vi "Send to DAQ - Core.vi"(6 "Timeout (ms)":i32=10000, 8 "error in (no error)":errorcluster, 9 "DAQ Message":T1, 10 "DAQ Address":cluster{"Port":u16, "Path":string}, 11 "DAQ Communication":refnum<class "DAQ Communication.lvclass">) -> (0 "error out":errorcluster)   [LabVIEW 2020, in "DAQ Sender.lvlib" / "DAQ Sender.lvclass"]
doc: "Use this VI to send data to the DAQ. If an entire file is needed to be sent, set File?=True and provide the path of the file to be sent in the Data field. DO NOT USE this VI from inside a uService."
uses:
  DAQ Sender.lvclass
  Interfaces/DAQ Communication/DAQ Communication.lvclass
  Interfaces/DAQ Communication/DAQ Message.ctl
  Ancestor/Ancestor/Ancestor.lvclass/Ancestor.ctl
  Support VIs/Circus Config Param - Core.vi
  Support VIs/Generate Error.vi
  Support VIs/Circus Root Path.vi
  FGV/Error Memory/Get Error Description.vi
  Support VIs/Get PC name.vi
  Ancestor/Ancestor/Read ID.vi
  Support VIs/Get Class Name.vi
  <vilib>/Utility/error.llb/Clear Errors.vi
  FGV/Error Memory/Error Memory Core.vi
  <vilib>/AdvancedString/Delimited String to 1D String Array.vi
  FGV/Error Memory/Error Crt Lvl checker.vi
  FGV/Error Memory/Error Memory Core.vi/40c8088d-b597-4017-91af-faa98e00292e.vi
  FGV/Error Memory/Error Memory Core.vi/d4a3ab98-063c-4e44-b43d-fbdcfe6c2be2.vi
  Support VIs/Global Constants.vi
  Support VIs/Global Memory.vi
  <vilib>/Utility/LVClass/Get LV Class Name.vi
  Support VIs/Is in Packed Library.vi
  Support VIs/TALOS Root path.vi
  Support VIs/Read CSV worksheet.vi
  <vilib>/Utility/error.llb/General Error Handler.vi
  <vilib>/Utility/config.llb/Open Config Data.vi
  <vilib>/Utility/config.llb/Get Section Names.vi
  <vilib>/Utility/config.llb/Get Key Names.vi
  <vilib>/Utility/config.llb/Read Key.vi
  <vilib>/Utility/config.llb/Read Key (String).vi
  <vilib>/Utility/config.llb/Close Config Data.vi
  Support VIs/Error Log.vi
  Ancestor/Ancestor/Ancestor.lvclass
  <vilib>/Comparison/Equal/Equal Functor/Equal Functor.lvclass
  TALOS.lvlib
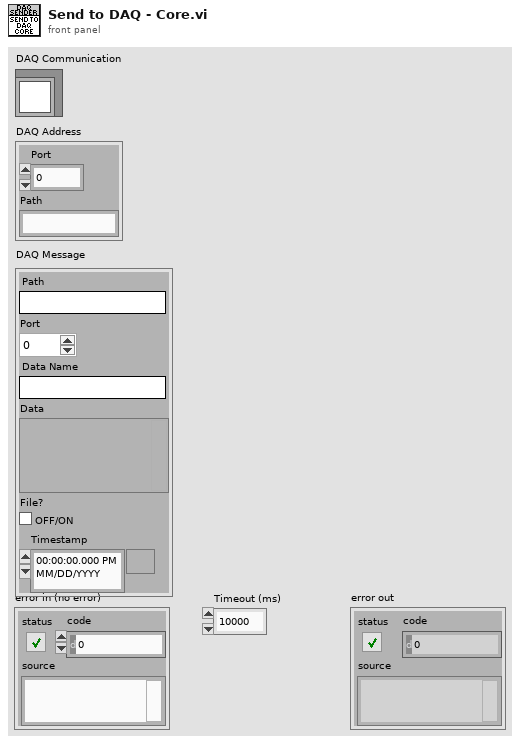
[diagram p1: front panel]
types:
  T1 = typedef "TALOS.lvlib/Interfaces.lvlib/DAQ Communication.lvclass/DAQ Message.ctl" = cluster{"Path":string, "Port":u16, "Data Name":string, "Data":variant, "File?":bool, "Timestamp":timestamp}
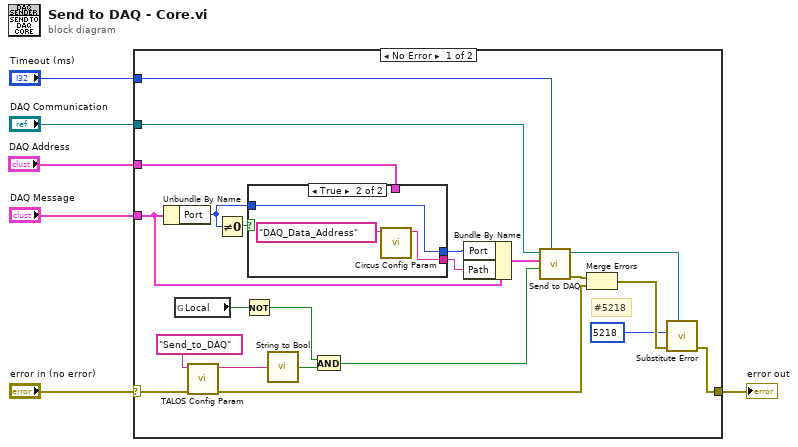
[diagram p0: block diagram]
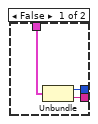
[diagram p2: hidden frame]
diagram:
  n1 = case shown="No Error" "error in (no error)" {
    selector: "error in (no error)" -> [w28 w35]
    tunnel: [w26 w35] -> w6
    tunnel: "Timeout (ms)" -> [w16 _]
    tunnel: "DAQ Communication" -> [w17 _]
    tunnel: "DAQ Address" -> [w20 _]
    tunnel: "DAQ Message" -> [w8 _]
    frame No Error {
      # "#5218"
      n2 = Unbundle By Name(w8) -> ("Port"=w9:u16)
      n3 = global read "Global Constants.vi" "Local"() -> (w25:bool)
      n4 = call "TALOS Config Param.vi"("error in (no error)"=w28, "Parameter Name"="Send_to_DAQ") -> ("error out"=w12:errorcluster, "Output"=w23:string)  [unwired: 8 in]
      n5 = Not Equal To 0?(x=w9) -> (x != 0?=w21:bool)
      n6 = Not(x=w25) -> (.not. x?=w24:bool)
      n7 = case shown="True" w21 {
        tunnel: [w31 w33] -> w18
        tunnel: [w30 w34] -> w19
        tunnel: w9 -> [_ w34]
        tunnel: w20 -> [w29 _]
        frame False {
          n8 = Unbundle(w29) -> ("Port"=w30:u16, "Path"=w31:string)
        }
        frame True {
          n9 = call "Circus Config Param.vi"("Parameter Name"="DAQ_Data_Address") -> ("Value"=w33:string)  [unwired: 9 in, 1 out]
        }
      }
      n10 = call "String to Bool.vi"("String"=w23) -> ("Boolean"=w22:bool)
      n11 = And(x=w24, y=w22) -> (x .and. y?=w14:bool)
      n12 = Bundle By Name(cluster=w8, "Port"=w19, "Path"=w18) -> (w10:T1)
      n13 = call-dynamic "Send to DAQ.vi"("Timeout (ms)"=w16, "Send to DAQ?"=w14, "DAQ Message"=w10, "DAQ Communication in"=w17) -> ("error out"=w13:errorcluster, "DAQ Communication out"=w15:refnum<class "DAQ Communication.lvclass">)  [unwired: 6 in]
      n14 = Merge Errors(w13, w12) -> (w11:errorcluster)
      n15 = call "Substitute Error.vi"("LabVIEW Object"=w15, "error in (no error)"=w11, "Error Code"=5218) -> ("error out"=w26:errorcluster)  [unwired: 8 in]
    }
    frame Error {
    }
  }
  "error out" <- w6
